vi "get_targets_simple.vi"(2 "error in (no error)":errorcluster, 3 "Remote Server Address":string="palantir") -> (0 "error out":errorcluster, 1 "Target Array":string[](array[string]))   [LabVIEW 2011]
uses:
  TCPdata.ctl
  TargetData.ctl
  CommonTargetData.ctl
panel:
  in  "CommonTargetData":T1
  in  "Target Array Type":T3(array[cluster])
  in  "Cluster":T4
  in  "Listen Port":u16=5311
  in  "Remote Server Port":u16=5310
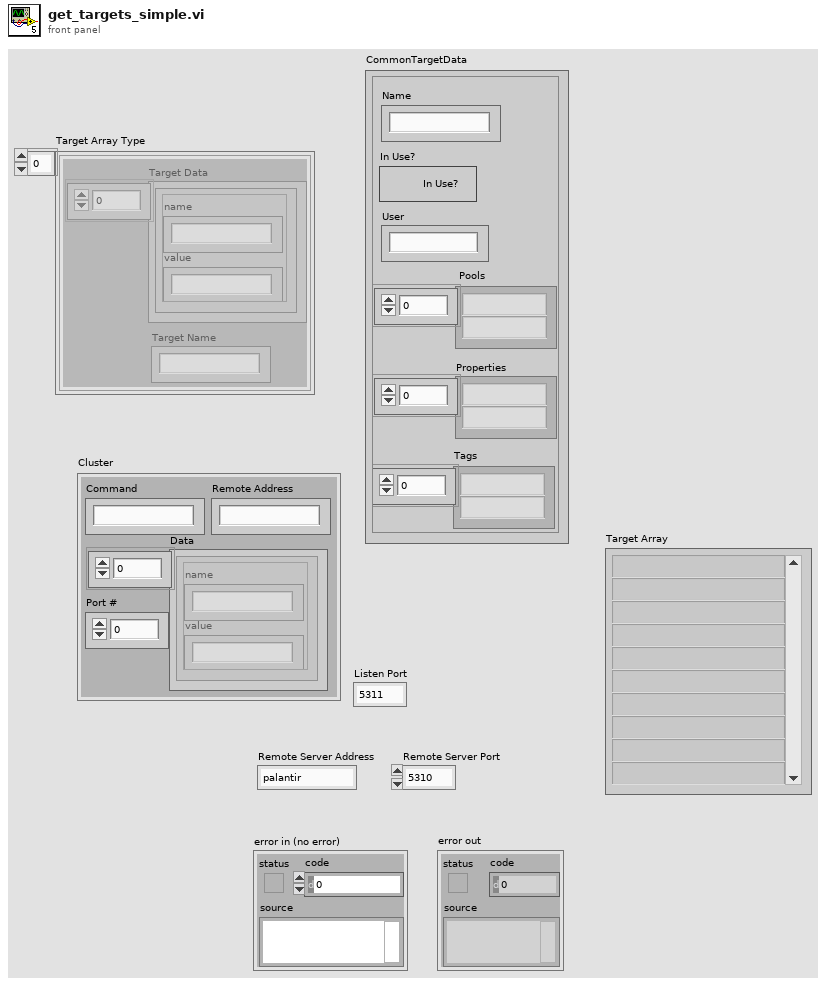
[diagram p1: front panel]
types:
  T1 = typedef "CommonTargetData.ctl" = cluster{"Name":string, "In Use?":bool, "User":string, " Pools":string[], "Tags":string[], "Properties":string[]}
  T2 = typedef "TargetData.ctl" = cluster{"name":string, "value":string}[]
  T3 = cluster{"Target Data":T2, "Target Name":string}[]
  T4 = typedef "TCPdata.ctl" = cluster{"Data":T2, "Command":string, "Remote Address":string, "Port #":u16}
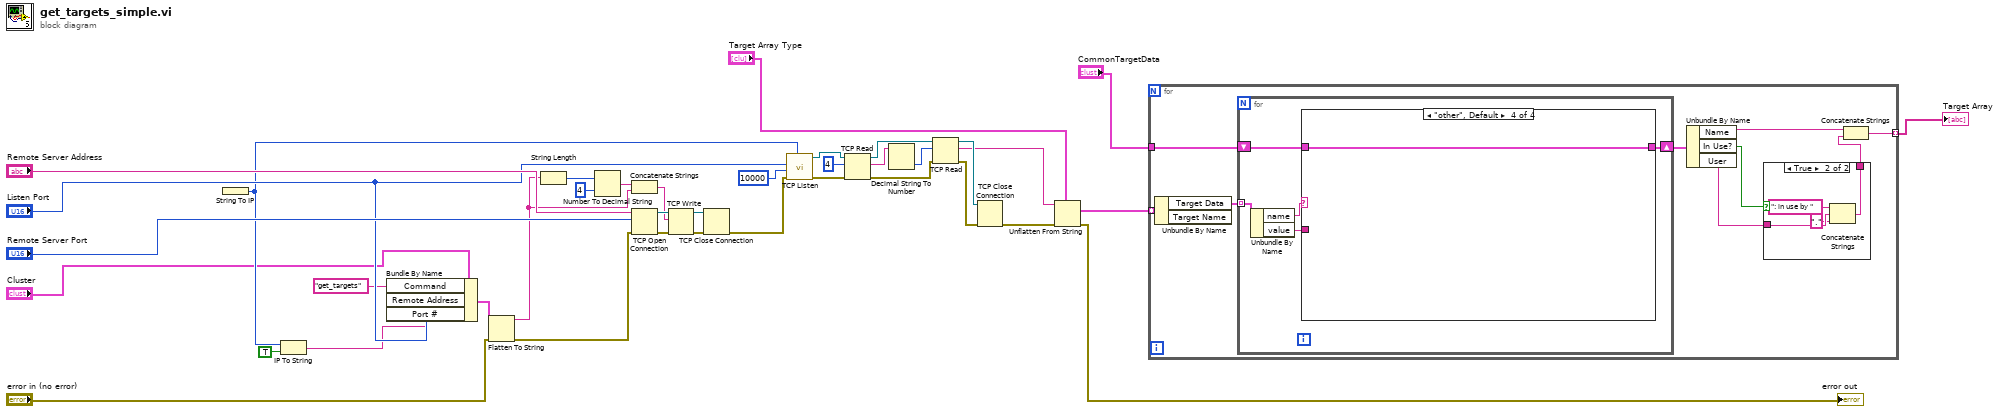
[diagram p0: block diagram]
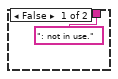
[diagram p2: hidden frame]
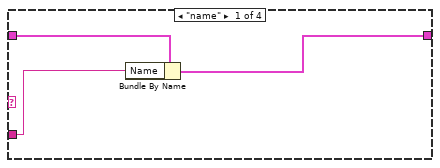
[diagram p3: hidden frame]
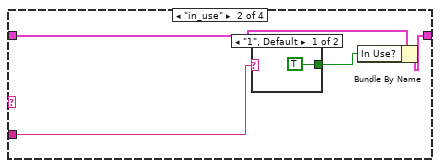
[diagram p4: hidden frame]
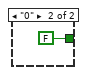
[diagram p5: hidden frame]
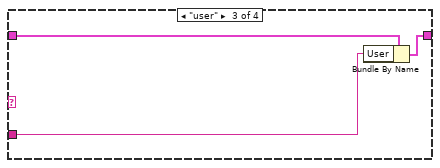
[diagram p6: hidden frame]
diagram:
  n1 = String To IP() -> (0:w24:u32)  [unwired: 1 in]
  n2 = IP To String(1:TRUE ("dot notation? (F)"), 2:w24) -> (0:w26:string)
  n3 = Bundle By Name(cluster="Cluster", "Command"="get_targets", "Remote Address"=w26, "Port #"="Listen Port") -> (w5:T4)
  n4 = Flatten To String(anything=w5, error in (no error)="error in (no error)") -> (data string=w19:string, error out=w17:errorcluster)  [unwired: 2 in, 1 out]
  n5 = String Length(string=w19) -> (length=w22:i32)
  n6 = Number To Decimal String(number=w22, width (-)=i16 4) -> (decimal integer string=w21:string)
  n7 = Concatenate Strings(w21, w19) -> (w23:string)
  n8 = TCP Open Connection(address="Remote Server Address", remote port or service name="Remote Server Port", error in (no error)=w17) -> (connection ID=w38:refnum<k5>, error out=w37:errorcluster)  [unwired: 2 out]
  n9 = TCP Write(connection ID=w38, data in=w23, error in (no error)=w37) -> (connection ID out=w35:refnum<k5>, error out=w36:errorcluster)  [unwired: 2 out]
  n10 = TCP Close Connection(connection ID=w35, error in (no error)=w36) -> (error out=w29:errorcluster)  [unwired: 2 out]
  n11 = call <vilib>:"TCP Listen.vi"("net address"=w24, "error in (no error)"=w29, "timeout ms (wait forever: -1)"=10000, "port"="Listen Port") -> ("error out"=w14:errorcluster, "connection ID"=w12:refnum<k5>)  [unwired: 3 in, 3 out]
  n12 = TCP Read(connection ID=w12, bytes to read=4, error in (no error)=w14) -> (connection ID out=w11:refnum<k5>, data out=w15:string, error out=w13:errorcluster)  [unwired: 1 in, 1 out]
  n13 = Decimal String To Number(string=w15) -> (number=w10:i32)  [unwired: 2 in, 1 out]
  n14 = TCP Read(connection ID=w11, bytes to read=w10, error in (no error)=w13) -> (connection ID out=w32:refnum<k5>, data out=w8:string, error out=w30:errorcluster)  [unwired: 1 in, 1 out]
  n15 = TCP Close Connection(connection ID=w32, error in (no error)=w30) -> (error out=w9:errorcluster)  [unwired: 2 out]
  n16 = Unflatten From String(type="Target Array Type", binary string=w8, error in (no error)=w9) -> (value=w6:T3, error out=→"error out":errorcluster)  [unwired: 2 in, 1 out]
  n17 = for {
    tunnel: w6 -> [w47] mode=indexing
    tunnel: "CommonTargetData" -> [w45]
    tunnel: [w39] -> w1 mode=indexing
    n18 = Unbundle By Name(w47) -> ("Target Data"=w46:T2)  [unwired: 1 out]
    n19 = for {
      tunnel: w46 -> [w57] mode=indexing
      shift-right: [w53] -> w44
      shift-left: w45 -> [w54]
      n20 = Unbundle By Name(w57) -> ("name"=w56:string, "value"=w55:string)
      n21 = case shown="\"other\", Default" w56 {
        tunnel: w55 -> [w58 w61 w67 _]
        tunnel: w54 -> [w60 w63 w69 w70]
        tunnel: [w59 w62 w68 w70] -> w53
        frame "name" {
          n22 = Bundle By Name(cluster=w60, "Name"=w58) -> (w59:T1)
        }
        frame "in_use" {
          n23 = case shown="\"1\", Default" w61 {
            tunnel: [TRUE ("In Use?") FALSE ("In Use?")] -> w64
            frame "1", Default {
            }
            frame "0" {
            }
          }
          n24 = Bundle By Name(cluster=w63, "In Use?"=w64) -> (w62:T1)
        }
        frame "user" {
          n25 = Bundle By Name(cluster=w69, "User"=w67) -> (w68:T1)
        }
        frame "other", Default {
        }
      }
    }
    n26 = Unbundle By Name(w44) -> ("Name"=w43:string, "In Use?"=w42:bool, "User"=w41:string)
    n27 = case shown="True" w42 {
      tunnel: w41 -> [_ w51]
      tunnel: [": not in use." w49] -> w40
      frame False {
      }
      frame True {
        n28 = Concatenate Strings(": in use by " ("string"), w51, "." ("string")) -> (w49:string)
      }
    }
    n29 = Concatenate Strings(w43, w40) -> (w39:string)
  }
  "Target Array" <- w1
